vi "CheckForStop.vi"(8 "Stop Button":bool, 9 "Miss":bool, 10 "Stop from main loop":bool) -> (0 "Stop output":T1)   [LabVIEW 2016]
panel:
  in  "Output cluster":T1
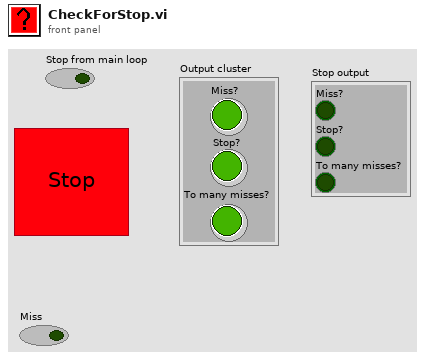
[diagram p1: front panel]
types:
  T1 = cluster{"Miss?":bool, "Stop?":bool, "To many misses?":bool}
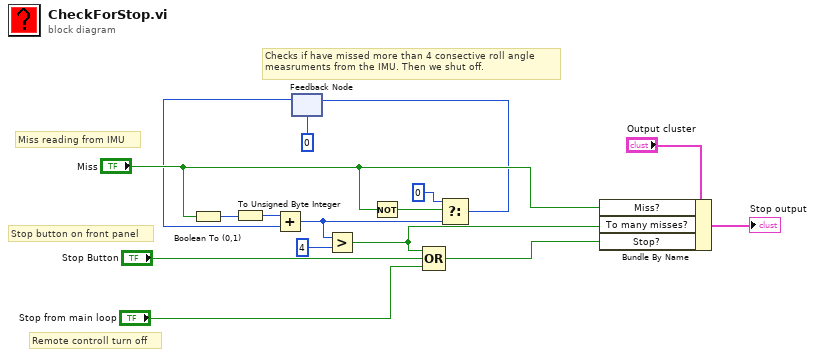
[diagram p0: block diagram]
diagram:
  # "Miss reading from IMU"
  # "Stop button on front panel"
  # "Remote controll turn off"
  # "Checks if have missed more than 4 consective roll angle\nmeasruments from the IMU. Then we shut off."
  n1 = Boolean To (0,1)(Boolean="Miss") -> (0, 1=w3:i16)
  n2 = To Unsigned Byte Integer(number=w3) -> (unsigned 8bit integer=w2:u8)
  n3 = feedback #1(u8 0 ("t")) -> (w6:u8)
  n4 = Add(x=w2, y=w6) -> (x+y=w10:u8)
  n5 = Greater?(x=w10, y=u8 4) -> (0:w12:bool)
  n6 = Not(x="Miss") -> (.not. x?=w8:bool)
  n7 = Compound Arithmetic op=OR(w12, "Stop Button", "Stop from main loop") -> (w13:bool)
  n8 = Select(t=u8 0, s=w8, f=w10) -> (s? t:f=w5:u8)
  n9 = feedback-in #1(w5) -> ()
  n10 = Bundle By Name(cluster="Output cluster", "Miss?"="Miss", "To many misses?"=w12, "Stop?"=w13) -> (→"Stop output":T1)
